vi "3.3.vi"() -> ()   [LabVIEW 2017]
panel:
  in  "长度（剩余） 2":i32
  in  "偏移量(0) 2":i32
  in  "长度（剩余）":i32
  in  "偏移量(0)":i32
  out "字符串 3":string
  in  "初始扫描位置":u32
  out "数值":dbl
  out "字符串 2":string
  in  "字符串":string
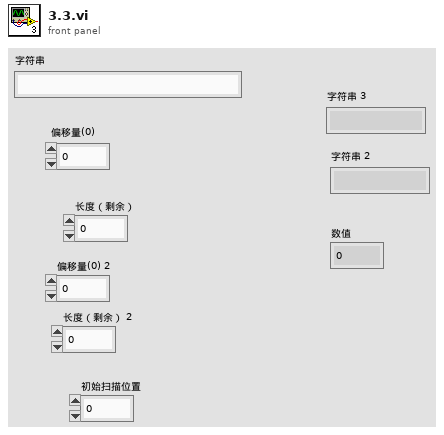
[diagram p1: front panel]
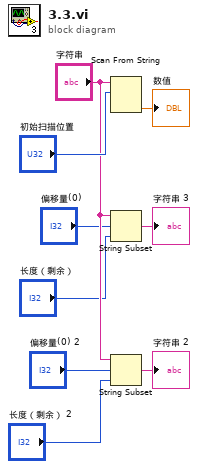
[diagram p0: block diagram]
diagram:
  n1 = Scan From String(input string="字符串", initial scan location="初始扫描位置") -> (output 1=→"数值":dbl)  [unwired: 3 in, 3 out]
  n2 = String Subset(string="字符串", offset (0)="偏移量(0)", length (rest)="长度（剩余）") -> (substring=→"字符串 3":string)
  n3 = String Subset(string="字符串", offset (0)="偏移量(0) 2", length (rest)="长度（剩余） 2") -> (substring=→"字符串 2":string)
